vi "PH_Stepmotor_BaseClass.get PSDB Axis ID.vi"(0 "i ref in":refnum<vi>, 5 "error in":errorcluster) -> (14 "i ref out":refnum<vi>, 19 "error out":errorcluster)   [LabVIEW 2014, in "PH_Stepmotor_BaseClass.lvlib"]
uses:
  PH_Stepmotor_BaseClass.lvlib
  PH_PSDBWriter/PH_PSDBWriter.PHELIX-Subsystems.ctl
  PH_PSDBWriter/PH_PSDBWriter.Data Status.ctl
  PH_PSDBWriter/PH_PSDBWriter.lvlib
  lib.lib/DimLVEvent/LVDimInterface/LVDimInterface.lvlib
panel:
  in  "PHELIX Subsysteme":T1 items=["Miscellaneous", "fs-Frontend", "ns-Frontend", "PreAmp", "MainAmp", "MAS", "COS", "Beamline", "Experiment Laserbay", "Experiment Laserlabor", "Experiment Z6", "Timing", "Pulsed Power"]
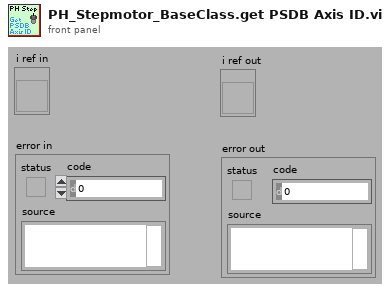
[diagram p1: front panel]
types:
  T1 = typedef "PH_PSDBWriter.lvlib/PH_PSDBWriter.PHELIX-Subsystems.ctl" = i32
  T2 = typedef "PH_Stepmotor_BaseClass.lvlib/PH_Stepmotor_BaseClass.i attribute.ctl" = cluster{"Device Error":errorcluster, "Axes PSDB Thread":cluster{"Ref":refnum<vi>, "Q-Ref":refnum<queue>, "Data Status":T3}, "Axes":T4[], "Axes PSDB Infos":cluster{"GUI Name":string, "PSDB Instance ID":i32, "PSDB Status Service ID":i32, "Axis":i32, "Class":string}[], "GUI Refs":T9}
  T3 = typedef "PH_PSDBWriter.lvlib/PH_PSDBWriter.Data Status.ctl" = i16
  T4 = typedef "PH_Stepmotor_BaseClass.lvlib/PH_Stepmotor_BaseClass.Axis Attributes.ctl" = cluster{"Settings":T5, "Endswitch?":bool, "DIM Service IDs":T7, "Activity":T8, "Configured?":bool, "Position":cluster{"Current":i32, "Target":i32}, "Position to set":cluster{"New?":bool, "Wanted":i32}, "Stop?":bool, "Reset?":bool, "Move?":bool, "Nothing connected?":bool}
  T5 = typedef "PH_Stepmotor_BaseClass.lvlib/PH_Stepmotor_BaseClass.Axis Settings.ctl" = cluster{"Sign change":bool, "Width":dbl, "Calibration":dbl, "Unit":string, "Motor Type":T6, "Unit Width":string, "Unit CF":string}
  T6 = typedef "PH_Stepmotor_BaseClass.lvlib/PH_Stepmotor_BaseClass.Motor Type.ctl" = enum16{"Unspecific", "OWIS 49.120.2633", "OWIS 49.060.1033", "OWIS 43.040.2558", "Diamond Motion 2200 series", "OWIS 49.120.266B.MV6", "Calorimeter", "Linear Stage 1", "MICOS VT-80", "MICOS VT-80 S", "Standa Rotstage nt0.95A", "PUF RA 320.200", "PUF RA 800.200", "PUF RA 800.400", "PUF RA 400.50", "1324.nn.800.50", "1324.n9c.800.50", "1324.nn.320.200", "1324.nn.400.200", "1324.nn.800.200", "1324.nn.400.50", "1324.8c9c.800.50", "1324.8c9c.400.200"}
  T7 = typedef "PH_Stepmotor_BaseClass.lvlib/PH_Stepmotor_BaseClass.Axis DIM Service IDs.ctl" = cluster{"Settings":i32, "Information":i32}
  T8 = typedef "PH_Stepmotor_BaseClass.lvlib/PH_Stepmotor_BaseClass.Axis Activity.ctl" = enum16{"No Information", "stopped", "running", "Failure", "Alarm", "stopped at backward ES", "stopped at foreward ES"}
  T9 = typedef "PH_Stepmotor_BaseClass.lvlib/PH_Stepmotor_BaseClass.GUI Refs.ctl" = cluster{"Axes Configuration":refnum<vi>, "Device Error":refnum<vi>, "Axes PSDB Infos":refnum<vi>}
  T10 = cluster{"GUI Name":string, "PSDB Instance ID":i32, "PSDB Status Service ID":i32, "Axis":i32, "Class":string}[]
  T11 = typedef "PH_PSDBWriter.lvlib/PH_PSDBWriter.i attribute.ctl" = cluster{"PSDB Status Service ID":i32, "Instance ID":i32, "Shot #":i32, "Subsystem":T1, "Data Status":T3, "Ref PSDB Status":refnum<vi>, "PSDB Error Code":i32, "PSDB Dataset":T12, "PSDB Thread":cluster{"Ref":refnum<vi>, "Q-Ref":refnum<queue>}, "PSDB Credentials":T20}
  T12 = typedef "PH_PSDBWriter.lvlib/PH_PSDBWriter.PSDB Dataset.ctl" = cluster{"Version":i32, "2D data Input":T13[], "Boolean Input":T15[], "Image Input":T16[], "Numeric Input":T18[], "String Input":T19[]}
  T13 = typedef "PH_PSDBWriter.lvlib/PH_PSDBWriter.2D dataset.ctl" = cluster{"name":string, "data":dbl[][], "axis description":T14}
  T14 = typedef "PSDB.lvlib/PSDB_AxisDescription.ctl" = cluster{"x axis label":string, "y axis label":string, "x axis unit":string, "y axis unit":string}
  T15 = typedef "PH_PSDBWriter.lvlib/PH_PSDBWriter.Boolean dataset.ctl" = cluster{"name":string, "data":bool, "unit":string}
  T16 = typedef "PH_PSDBWriter.lvlib/PH_PSDBWriter.Image dataset.ctl" = cluster{"name":string, "data":T17, "unit":string}
  T17 = typedef "IMAQ Image.ctl" = refnum<image>
  T18 = typedef "PH_PSDBWriter.lvlib/PH_PSDBWriter.Numeric dataset.ctl" = cluster{"name":string, "data":dbl, "unit":string}
  T19 = typedef "PH_PSDBWriter.lvlib/PH_PSDBWriter.String dataset.ctl" = cluster{"name":string, "data":string, "unit":string}
  T20 = typedef "PH_Common.lvlib/PH_Connection.PSDB Credentials.ctl" = cluster{"PW":string, "ID":string, "DS":string}
  T21 = cluster{"GUI Name":string, "Class":string, string}
  T22 = cluster{"GUI Name":string, "PSDB Instance ID":i32, "PSDB Status Service ID":i32, "Axis":i32, "Class":string}
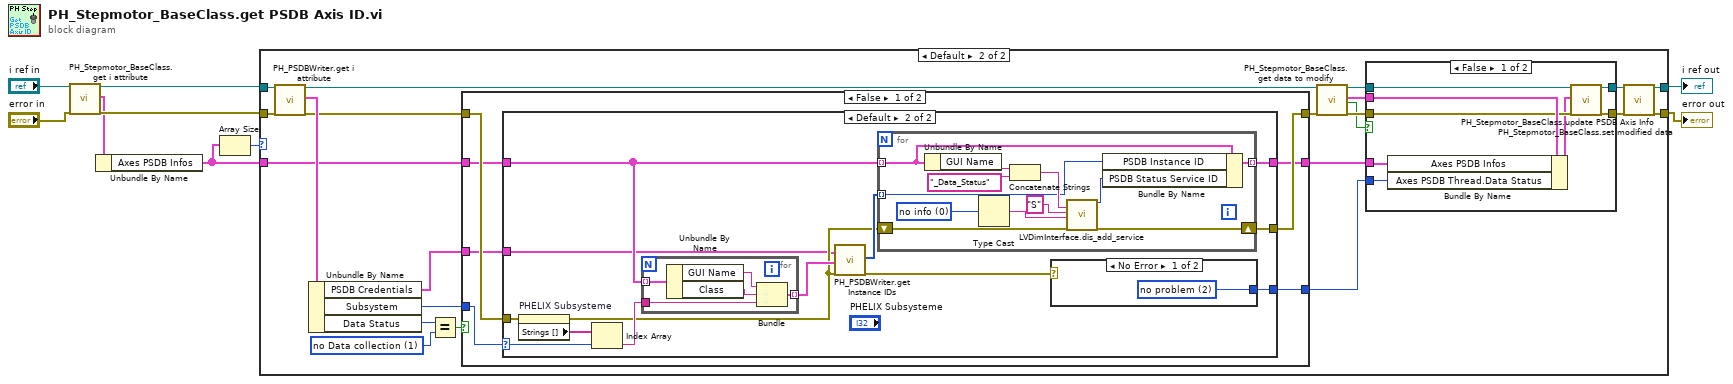
[diagram p0: block diagram]
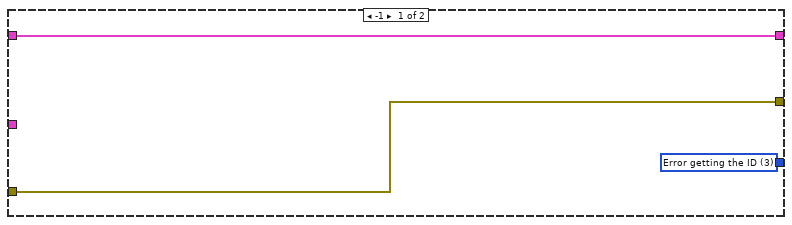
[diagram p3: hidden frame]
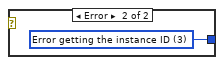
[diagram p4: hidden frame]
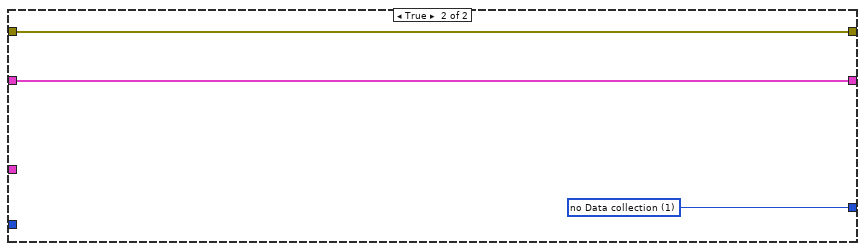
[diagram p5: hidden frame]
diagram:
  n1 = call "PH_Stepmotor_BaseClass.get i attribute.vi"("i ref in"="i ref in", "error in (no error)"="error in") -> ("i ref out"=w4:refnum<vi>, "i attribute"=w3:T2, "error out"=w5:errorcluster)  [unwired: 15 in]
  n2 = Unbundle By Name(w3) -> ("Axes PSDB Infos"=w2:T10)
  n3 = Array Size(array=w2) -> (size(s)=w1:i32)
  n4 = case shown="Default" w1 {
    tunnel: [w11 w33] -> w9
    tunnel: [w10 w32] -> w8
    tunnel: w5 -> [w10 w31]
    tunnel: w4 -> [w11 w30]
    tunnel: w2 -> [_ w16]
    frame 0 {
    }
    frame Default {
      w21 = T3 1 items=["no info", "no Data collection", "no problem", "Error getting the instance ID", "Error writing Data to data base"] ("Metadata.Data Status")
      n5 = call "PH_PSDBWriter.get i attribute.vi"("i ref in"=w30, "error in (no error)"=w31) -> ("i ref out"=w13:refnum<vi>, "i attribute"=w19:T11, "error out"=w17:errorcluster)  [unwired: 15 in]
      n6 = Unbundle By Name(w19) -> ("PSDB Credentials"=w12:T20, "Subsystem"=w18:T1, "Data Status"=w20:T3)
      n7 = Equal?(x=w20, y=w21) -> (x = y?=w14:bool)
      n8 = case shown="False" w14 {
        tunnel: [w40 w77] -> w25
        tunnel: [w39 w76] -> w22
        tunnel: w18 -> [w35 _]
        tunnel: w17 -> [w38 w77]
        tunnel: w16 -> [w37 w76]
        tunnel: [w36 w78] -> w15
        tunnel: w12 -> [w34 _]
        frame False {
          n9 = case shown="Default" w35 {
            selector: w35 -> [_ w45]
            tunnel: [w43 w56] -> w40
            tunnel: [w42 w55] -> w39
            tunnel: w38 -> [w43 w53]
            tunnel: w37 -> [w42 w52]
            tunnel: [w41 w48] -> w36
            tunnel: w34 -> [_ w44]
            frame -1 {
              w41 = T3 3 items=["no info", "no Data collection", "no problem", "Error getting the ID", "Error writing Data", "Error getting the subsystem", "Error getting the Shot ID", "Error getting the Shot Types", "Error getting the Experiments", "Error verifying wanted Shottype", "Error verifying wanted Experiment"] ("Metadata.Data Status")
            }
            frame Default {
              n10 = property on="PHELIX Subsysteme" class="Ring (strict)"(error in=w53) -> (error out=w46:errorcluster, "Strings []"=w54:string[])  [unwired: 1 in, 1 out]
              n11 = Index Array(array=w54, index=w45) -> (element=w51:string)
              n12 = for {
                tunnel: w52 -> [w63] mode=indexing
                tunnel: w51 -> [w60]
                tunnel: [w59] -> w50 mode=indexing
                n13 = Unbundle By Name(w63) -> ("GUI Name"=w62:string, "Class"=w61:string)
                n14 = Bundle("GUI Name"=w62, "Class"=w61, w60) -> (w59:T21)  [unwired: 1 in]
              }
              n15 = call "PH_PSDBWriter.get Instance IDs.vi"("PSDB Credentials"=w44, "Instances"=w50, "error in"=w46) -> ("Instance IDs"=w47:i32[], "error out"=w49:errorcluster)  [unwired: 15 in]
              n16 = for {
                tunnel: w52 -> [w65] mode=indexing
                shift-right: [w74] -> w56
                shift-left: w46 -> [w75]
                tunnel: [w72] -> w55 mode=indexing
                tunnel: w47 -> [w64] mode=indexing
                w66 = T3 0 items=["no info", "no Data collection", "no problem", "Error getting the instance ID", "Error writing Data to data base"] ("Metadata.Data Status")
                n17 = Unbundle By Name(w65) -> ("GUI Name"=w71:string)
                n18 = Type Cast(x=w66) -> (*(type *) &x=w67:string)  [unwired: 1 in]
                n19 = Concatenate Strings(w71, "_Data_Status" ("string")) -> (w69:string)
                n20 = call "LVDimInterface.dis_add_service.vi"("serviceName"=w69, "typeDescriptor"="S", "data"=w67, "error in (no error)"=w75) -> ("my_serviceID"=w73:i32, "error out"=w74:errorcluster)  [unwired: 14 in]
                n21 = Bundle By Name(cluster=w65, "PSDB Instance ID"=w64, "PSDB Status Service ID"=w73) -> (w72:T22)
              }
              n22 = case shown="No Error" w49 {
                tunnel: [w57 w58] -> w48
                frame No Error {
                  w57 = T3 2 items=["no info", "no Data collection", "no problem", "Error getting the instance ID", "Error writing Data to data base"] ("Metadata.Data Status")
                }
                frame Error {
                  w58 = T3 3 items=["no info", "no Data collection", "no problem", "Error getting the instance ID", "Error writing Data to data base"] ("Metadata.Data Status")
                }
              }
            }
          }
        }
        frame True {
          w78 = T3 1 items=["no info", "no Data collection", "no problem", "Error getting the ID", "Error writing Data", "Error getting the subsystem", "Error getting the Shot ID", "Error getting the Shot Types", "Error getting the Experiments", "Error verifying wanted Shottype", "Error verifying wanted Experiment"] ("Metadata.Data Status")
        }
      }
      n23 = call "PH_Stepmotor_BaseClass.get data to modify.vi"("i ref in"=w13, "error in (no error)"=w25) -> ("i ref out"=w27:refnum<vi>, "i attribute"=w26:T2, "timed out"=w23:bool, "error out"=w24:errorcluster)  [unwired: 14 in]
      n24 = case shown="False" w23 {
        tunnel: [w86 w88] -> w29
        tunnel: [w85 w87] -> w28
        tunnel: w27 -> [w84 w88]
        tunnel: w26 -> [w83 _]
        tunnel: w24 -> [w82 w87]
        tunnel: w22 -> [w80 _]
        tunnel: w15 -> [w79 _]
        frame False {
          n25 = Bundle By Name(cluster=w83, "Axes PSDB Infos"=w80, "Axes PSDB Thread.Data Status"=w79) -> (w81:T2)
          n26 = call "PH_Stepmotor_BaseClass.set modified data.vi"("i ref in"=w84, "i attribute"=w81, "error in (no error)"=w82) -> ("i ref out"=w86:refnum<vi>, "error out"=w85:errorcluster)  [unwired: 15 in]
        }
        frame True {
        }
      }
      n27 = call "PH_Stepmotor_BaseClass.update PSDB Axis Info.vi"("i ref in"=w29, "error in"=w28) -> ("i ref out"=w33:refnum<vi>, "error out"=w32:errorcluster)  [unwired: 16 in]
    }
  }
  "error out" <- w8
  "i ref out" <- w9
